vi "CTL_PropCtlr.vi"(6 "Pump Speed":T1=enum."SLOW", 8 "Empty Inches":dbl, 9 "Full Inches":dbl, 10 "Level PV":dbl, 11 "Level SP":dbl) -> (1 "Pump Speed Out":T1, 2 "X< Neg":bool, 3 "X>Pos":bool, 5 "Neg <X<Pos":bool)   [LabVIEW 2024]
uses:
  Control Definitions/Def_PumpSpeed.ctl
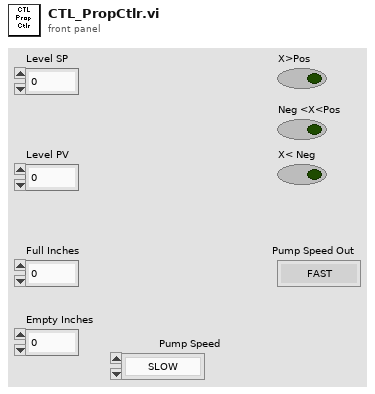
[diagram p1: front panel]
types:
  T1 = typedef "Def_PumpSpeed.ctl" = enum16{"FAST", "SLOW", "CREEP", "STOP"}
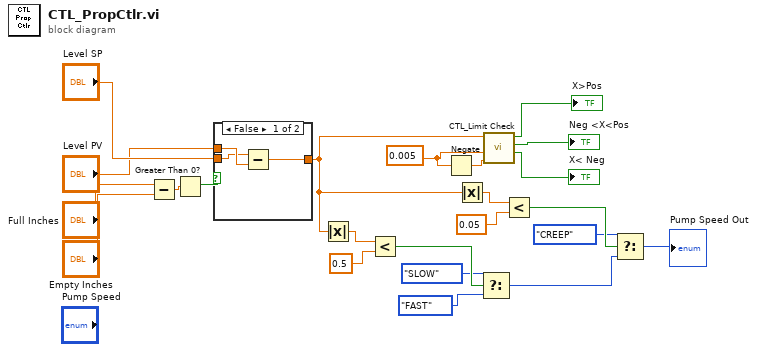
[diagram p0: block diagram]
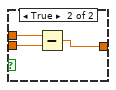
[diagram p2: hidden frame]
diagram:
  w13 = 0.005 ("Pos Limit")
  n1 = Subtract(x="Full Inches", y="Empty Inches") -> (x-y=w19:dbl)
  n2 = Greater Than 0?(x=w19) -> (x > 0?=w20:bool)
  n3 = case shown="False" w20 {
    tunnel: [w24 w29] -> w5
    tunnel: "Level PV" -> [w26 w28]
    tunnel: "Level SP" -> [w25 w27]
    frame False {
      n4 = Subtract(x=w25, y=w26) -> (x-y=w24:dbl)
    }
    frame True {
      n5 = Subtract(x=w28, y=w27) -> (x-y=w29:dbl)
    }
  }
  n6 = Absolute Value(x=w5) -> (abs(x)=w21:dbl)
  n7 = Less?(x=w21, y=0.5) -> (x < y?=w23:bool)
  n8 = Negate(x=w13) -> (-x=w11:dbl)
  n9 = Absolute Value(x=w5) -> (abs(x)=w6:dbl)
  n10 = Select(t=Def_PumpSpeed."SLOW" ("Pump Speed"), s=w23, f=Def_PumpSpeed."FAST") -> (s? t:f=w2:T1)
  n11 = call "CTL_Limit Check.vi"("Neg Limit"=w11, "Pos Limit"=w13, "X"=w5) -> ("X< Neg"=→"X< Neg":bool, "Neg <X<Pos"=→"Neg <X<Pos":bool, "X>Pos"=→"X>Pos":bool)  [unwired: 6 in]
  n12 = Less?(x=w6, y=0.05) -> (x < y?=w9:bool)
  n13 = Select(t=Def_PumpSpeed."CREEP" ("Pump Speed"), s=w9, f=w2) -> (s? t:f=→"Pump Speed Out":T1)
